vi "setRunModeSubVi.vi"(5 "variables":string[][](array[string]), 6 "Arguments":string, 7 "UDP message":string, 8 "user error":errorcluster, 9 "config array":string[][](array[string])) -> (0 "USER error out":errorcluster, 1 "UDP message out":string, 2 "variables out":string[][](array[string]), 3 "String 2":string, 4 "RunMode":bool)   [LabVIEW 2013]
panel:
  in  "RunMode in":bool
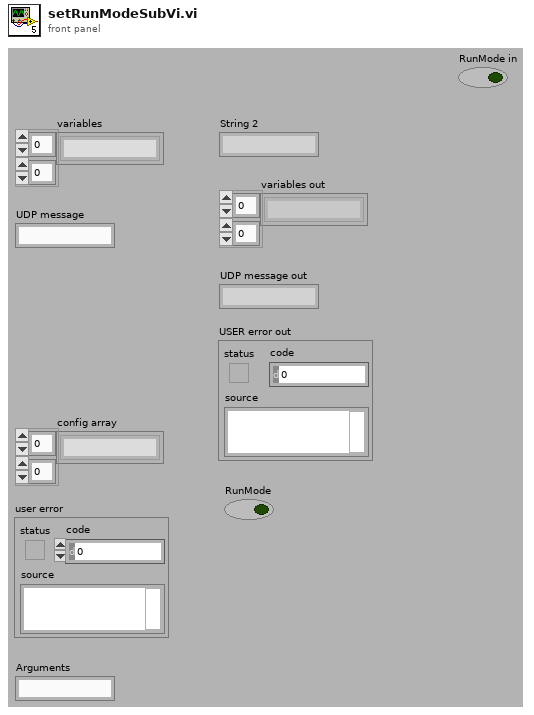
[diagram p1: front panel]
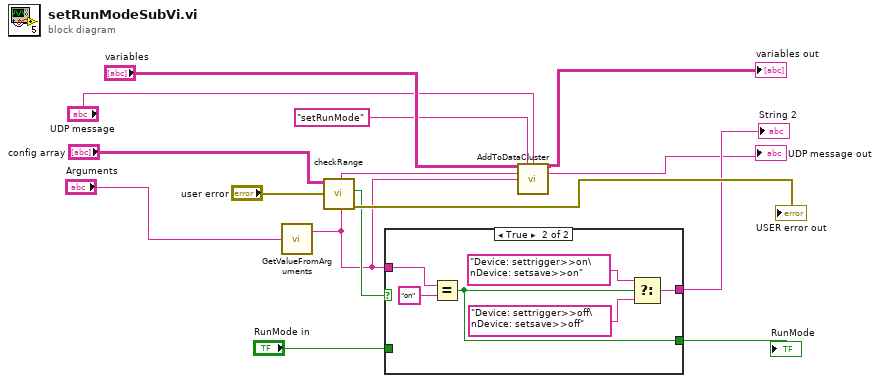
[diagram p0: block diagram]
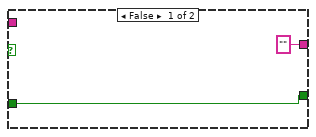
[diagram p2: hidden frame]
diagram:
  n1 = call "GetValueFromArguments.vi"("Arguments"="Arguments") -> ("setValue"=w2:string)  [unwired: 1 out]
  n2 = call "checkRange.vi"("USER error in"="user error", "config array"="config array") -> ("USER error out"=→"USER error out":errorcluster, "OK to change"=w11:bool)  [unwired: 3 in, 1 out]
  n3 = case shown="True" w11 {
    tunnel: ["" w19] -> w9
    tunnel: w2 -> [_ w18]
    tunnel: [w15 w17] -> w13
    tunnel: "RunMode in" -> [w15 _]
    frame False {
    }
    frame True {
      n4 = Equal?(x=w18, y="on") -> (x = y?=w17:bool)
      n5 = Select(t="Device: settrigger>>on\nDevice: setsave>>on", s=w17, f="Device: settrigger>>off\nDevice: setsave>>off") -> (s? t:f=w19:string)
    }
  }
  "RunMode" <- w13
  "String 2" <- w9
  n6 = call "AddToDataCluster.vi"("variables"="variables", "command"="setRunMode" ("String"), "UDP message"="UDP message", "set value"=w2, "actual value"=w2) -> ("variables out"=→"variables out":string[][], "UDP message out"=→"UDP message out":string)  [unwired: 8 in, 1 out]
